vi "Env.vi"(0 "Name":string, 1 "Value In":variant) -> (2 "Value Out":variant, 3 "names":string[](array[string]), 4 "values":variant[](array[variant]))   [LabVIEW 2014]
uses:
  Env.global.vi
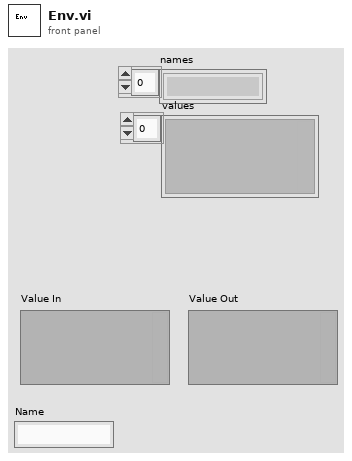
[diagram p1: front panel]
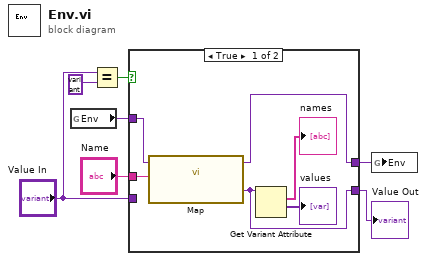
[diagram p0: block diagram]
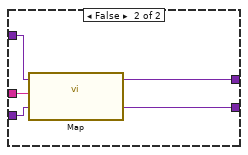
[diagram p2: hidden frame]
diagram:
  n1 = global read "Env.global.vi" "Env"() -> (w4:variant)
  n2 = Equal?(x="Value In", y=variant ("Value In")) -> (x = y?=w6:bool)
  n3 = case shown="True" w6 {
    tunnel: [w11 w18] -> w1
    tunnel: "Value In" -> [_ w17]
    tunnel: w4 -> [w13 w16]
    tunnel: "Name" -> [w12 w15]
    tunnel: [w10 w14] -> w2
    frame True {
      n4 = call "Map.vi"("Name"=w12, "Map In"=w13) -> ("Value Out"=w10:variant, "Map Out"=w11:variant)  [unwired: 1 in]
      n5 = Get Variant Attribute(Variant=w10) -> (names=→"names":string[], values=→"values":variant[])  [unwired: 3 in, 2 out]
    }
    frame False {
      n6 = call "Map.vi"("Value In"=w17, "Name"=w15, "Map In"=w16) -> ("Value Out"=w14:variant, "Map Out"=w18:variant)
    }
  }
  "Value Out" <- w2
  n7 = global write "Env.global.vi" "Env"(w1) -> ()
